vi "PlayQueue.vi"(0 "Program Interface in":refnum<class "Program Interface.lvclass">, 1 "robot":refnum<class "Universal Robot.lvclass">, 5 "error in (no error)":errorcluster) -> (14 "Program Interface out":refnum<class "Program Interface.lvclass">, 19 "error out":errorcluster)   [LabVIEW 2016, in "Program Interface.lvclass"]
uses:
  Program Interface.lvclass
  Universal Robot/Universal Robot.lvclass
  Program Interface.lvclass/Program Interface.ctl
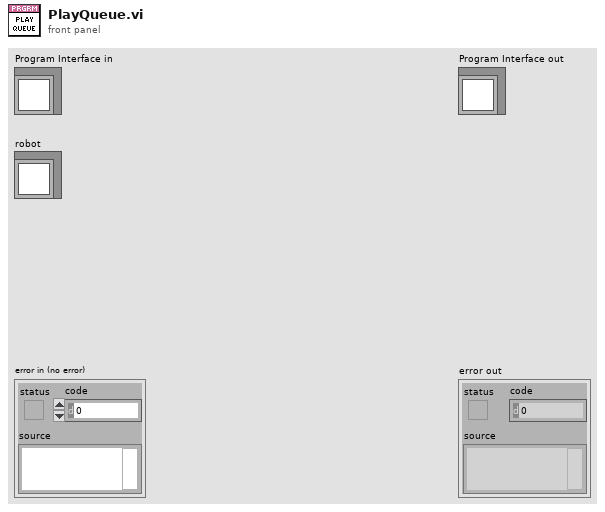
[diagram p1: front panel]
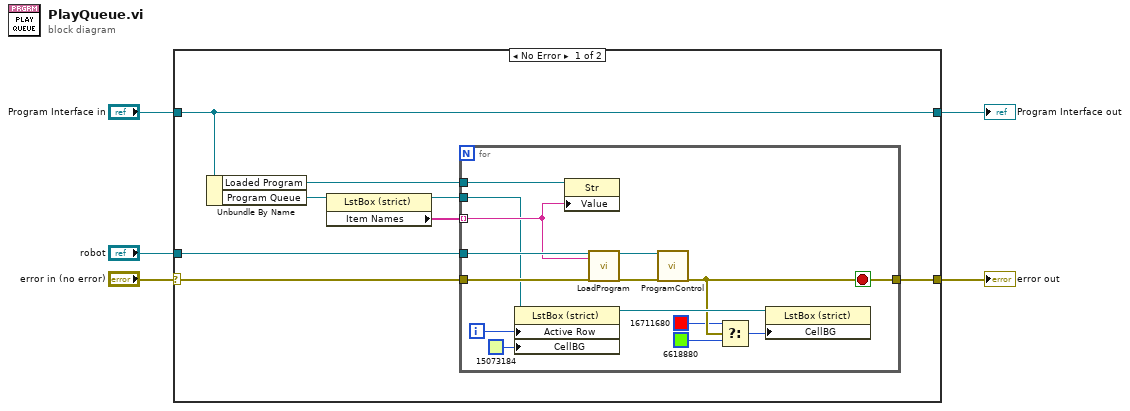
[diagram p0: block diagram]
diagram:
  n1 = case shown="No Error" "error in (no error)" {
    selector: "error in (no error)" -> [w12 w29]
    tunnel: [w11 w29] -> w4
    tunnel: [w13 w28] -> w2
    tunnel: "Program Interface in" -> [w13 w28]
    tunnel: "robot" -> [w8 _]
    frame No Error {
      n2 = Unbundle By Name(w13) -> ("Loaded Program"=w7:refnum<vi>, "Program Queue"=w10:refnum<vi>)
      n3 = property class="LstBox (strict)"(reference=w10) -> (reference out=w6:refnum<vi>, "Item Names"=w9:string[])  [unwired: 1 in, 1 out]
      n4 = for {
        tunnel: w9 -> [w23] mode=indexing
        tunnel: w8 -> [w25]
        tunnel: w12 -> [w27]
        tunnel: [w18] -> w11
        tunnel: w7 -> [w24]
        tunnel: w6 -> [w22]
        i -> [w21]
        stop <- w18 stop-if-true
        n5 = property class="LstBox (strict)"(reference=w22, "Active Row"=w21, "CellBG"=u32 15073184) -> (reference out=w19:refnum<vi>)  [unwired: 1 in, 1 out]
        n6 = property class="Str"(reference=w24, "Value"=w23) -> ()  [unwired: 1 in, 2 out]
        n7 = call-dynamic "LoadProgram.vi"("Universal Robot.lvclass in"=w25, "program"=w23, "error in (no error)"=w27) -> ("Universal Robot.lvclass out"=w26:refnum<class "Universal Robot.lvclass">, "error out"=w14:errorcluster)  [unwired: 15 in]
        n8 = call-dynamic "ProgramControl.vi"("Universal Robot.lvclass in"=w26, "error in (no error)"=w14) -> ("error out"=w18:errorcluster)  [unwired: 15 in, 2 out]
        n9 = Select(t=u32 16711680, s=w18, f=u32 6618880) -> (s? t:f=w15:u32)
        n10 = property class="LstBox (strict)"(reference=w19, "CellBG"=w15) -> ()  [unwired: 1 in, 2 out]
      }
    }
    frame Error {
    }
  }
  "error out" <- w4
  "Program Interface out" <- w2
